vi "Connect.vi"(8 "error in (no error)":errorcluster, 11 "IVI Oscilloscope in":refnum<class "IVI Oscilloscope.lvclass">) -> (0 "error out":errorcluster, 3 "IVI Oscilloscope out":refnum<class "IVI Oscilloscope.lvclass">)   [LabVIEW 2014, in "IVI Oscilloscope.lvclass"]
uses:
  IVI Oscilloscope.lvclass
  IVI Oscilloscope.lvclass/IVI Oscilloscope.ctl
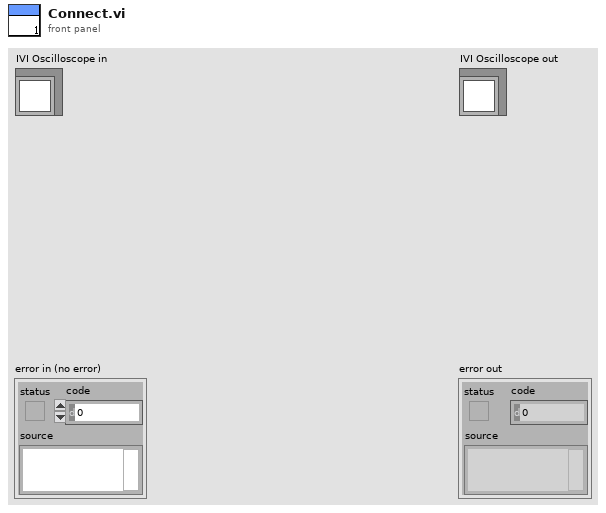
[diagram p1: front panel]
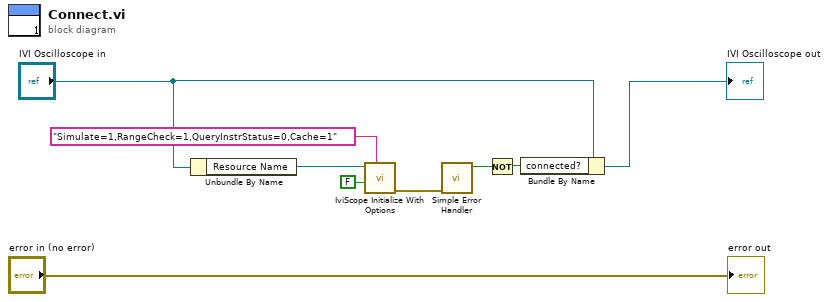
[diagram p0: block diagram]
diagram:
  n1 = Unbundle By Name("IVI Oscilloscope in") -> ("Resource Name"=w2:refnum<k15>)
  n2 = call <vilib>:"IviScope Initialize With Options.vi"("option string (\"Simulate=0,RangeCheck=1,QueryInstrStatus=0,Cache=1\")"="Simulate=1,RangeCheck=1,QueryInstrStatus=0,Cache=1" ("option string (\"Simulate=0,RangeCheck=1,QueryInstrStatus=0,Cache=1\")"), "reset device (True)"=FALSE, "logical name (\"SampleScope\")"=w2) -> ("error out"=w7:errorcluster)  [unwired: 7 in, 1 out]
  n3 = call <vilib>:"Simple Error Handler.vi"("error in (no error)"=w7) -> ("error?"=w6:bool)  [unwired: 4 in, 4 out]
  n4 = Not(x=w6) -> (.not. x?=w3:bool)
  n5 = Bundle By Name(cluster="IVI Oscilloscope in", "connected?"=w3) -> (→"IVI Oscilloscope out":refnum<class "IVI Oscilloscope.lvclass">)
  "error out" <- "error in (no error)"
